vi "_PC_Pub calc_linspace.vi"(7 "split_items":i32=7, 10 "min_val":dbl=-5.0 format="%#_13g", 11 "max_val":dbl=5.0 format="%#_13g") -> (3 "new data":dbl[](array[numeric]))   [LabVIEW 2018]
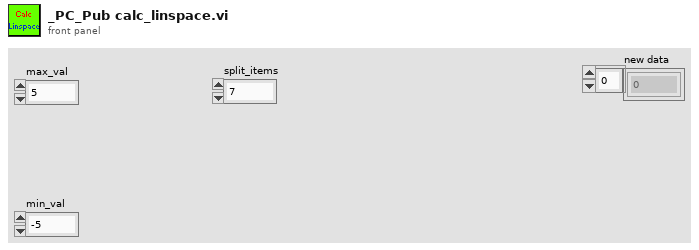
[diagram p1: front panel]
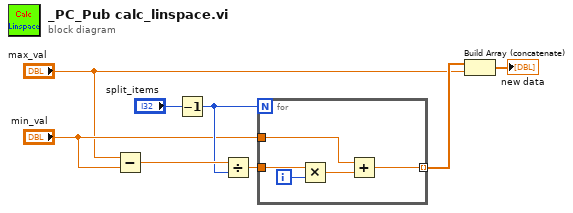
[diagram p0: block diagram]
diagram:
  n1 = Subtract(x="max_val", y="min_val") -> (x-y=w7:dbl)
  n2 = Decrement(x="split_items") -> (x-1=w6:i32)
  n3 = Divide(x=w7, y=w6) -> (x/y=w4:dbl)
  n4 = for {
    N: w6 -> [_]
    tunnel: "min_val" -> [w10]
    tunnel: w4 -> [w13]
    tunnel: [w9] -> w3 mode=indexing
    i -> [w12]
    n5 = Multiply(x=w13, y=w12) -> (x*y=w11:dbl)
    n6 = Add(x=w10, y=w11) -> (x+y=w9:dbl)
  }
  n7 = Build Array (concatenate)(w3, "max_val") -> (→"new data":dbl[])
